vi "readFromXML.vi"(8 "error in (no error)":errorcluster, 10 "XML in":string="<ClockTimes>\n<hours>1.112</hours>\n<minutesTime>2.223</minutesTime>\n<secondsTime>3.334</secondsTime>\n</ClockTimes>", 11 "ClockTimes in":refnum<class "ClockTimes.lvclass">) -> (0 "error out":errorcluster, 3 "ClockTimes out":refnum<class "ClockTimes.lvclass">)   [LabVIEW 2014, in "TCSDataDefinitions.lvlib" / "TCSPublicStatus.lvlib" / "CurrentTimes.lvlib" / "ClockTimes.lvclass"]
uses:
  ClockTimes.lvclass
  <userlib>/Common/UnitsAndXML/FlattenItemWithUnitToXML/FlattenTimeToXML/TimeUnit.ctl
  ClockTimes.lvclass/ClockTimes.ctl
  <userlib>/Common/UnitsAndXML/UnitsAndXML.lvlib
  <userlib>/Common/XML/XMLParser/XMLParser.lvclass
panel:
  out "seconds":dbl[unit]=3.334
  out "minutes":dbl[unit]=133.38
  out "hours":dbl[unit]=4003.2000000000003
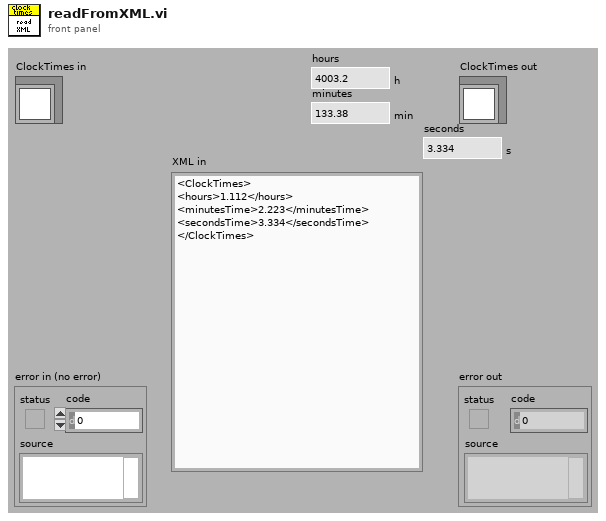
[diagram p1: front panel]
types:
  T1 = typedef "UnitsAndXML.lvlib/TimeUnit.ctl" = enum16{"s", "d", "h", "min", "a"}
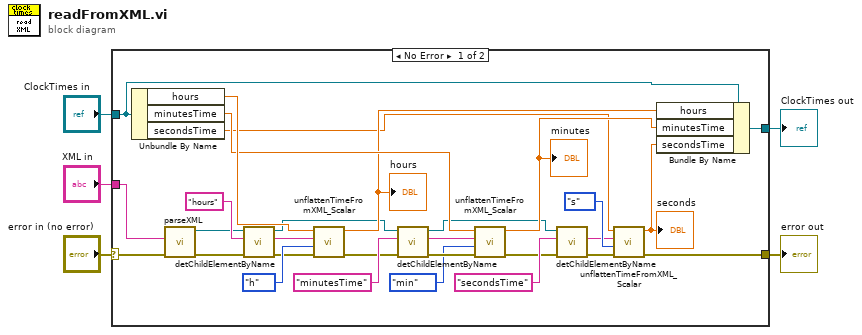
[diagram p0: block diagram]
diagram:
  n1 = case shown="No Error" "error in (no error)" {
    selector: "error in (no error)" -> [w13 w36]
    tunnel: [w12 w36] -> w4
    tunnel: [w23 w35] -> w2
    tunnel: "ClockTimes in" -> [w24 w35]
    tunnel: "XML in" -> [w33 _]
    frame No Error {
      n2 = Unbundle By Name(w24) -> ("hours"=w30:dbl[unit], "minutesTime"=w25:dbl[unit], "secondsTime"=w10:dbl[unit])
      n3 = call <userlib>:"parseXML.vi"("error in (no error)"=w13, "XMLString in"=w33) -> ("error out"=w34:errorcluster, "Element out"=w8:refnum<class "XMLParser.lvclass">)  [unwired: 8 in]
      n4 = call <userlib>:"detChildElementByName.vi"("error in (no error)"=w34, "childName"="hours" ("ChildName"), "Element in"=w8) -> ("error out"=w28:errorcluster, "childXML"=w31:string, "Element out"=w7:refnum<class "XMLParser.lvclass">)  [unwired: 5 in, 1 out]
      n5 = call <userlib>:"unflattenTimeFromXML_Scalar.vi"("error in (no error)"=w28, "timeUnitInXML"=TimeUnit."h", "xmlString"=w31, "timeForType"=w30) -> ("error out"=w20:errorcluster, "time"=w21:dbl[unit])  [unwired: 6 in]
      "hours" <- w21
      n6 = call <userlib>:"detChildElementByName.vi"("error in (no error)"=w20, "childName"="minutesTime" ("ChildName"), "Element in"=w7) -> ("error out"=w19:errorcluster, "childXML"=w26:string, "Element out"=w6:refnum<class "XMLParser.lvclass">)  [unwired: 5 in, 1 out]
      n7 = call <userlib>:"unflattenTimeFromXML_Scalar.vi"("error in (no error)"=w19, "timeUnitInXML"=TimeUnit."min", "xmlString"=w26, "timeForType"=w25) -> ("error out"=w15:errorcluster, "time"=w22:dbl[unit])  [unwired: 6 in]
      "minutes" <- w22
      n8 = call <userlib>:"detChildElementByName.vi"("error in (no error)"=w15, "childName"="secondsTime" ("ChildName"), "Element in"=w6) -> ("error out"=w14:errorcluster, "childXML"=w9:string)  [unwired: 5 in, 2 out]
      n9 = call <userlib>:"unflattenTimeFromXML_Scalar.vi"("error in (no error)"=w14, "timeUnitInXML"=TimeUnit."s", "xmlString"=w9, "timeForType"=w10) -> ("error out"=w12:errorcluster, "time"=w11:dbl[unit])  [unwired: 6 in]
      "seconds" <- w11
      n10 = Bundle By Name(cluster=w24, "hours"=w21, "minutesTime"=w22, "secondsTime"=w11) -> (w23:refnum<class "ClockTimes.lvclass">)
    }
    frame Error {
    }
  }
  "error out" <- w4
  "ClockTimes out" <- w2
